vi "SMTP Email Convert Recipients UTF-8.vi"(0 "recipients":string[](array[string]), 1 "error in":errorcluster) -> (2 "convertible recipients":string[](array[string]), 3 "unconvertible recipients":string[](array[string]), 4 "error out":errorcluster)   [LabVIEW 2011, in "NewNI_SMTPEmail.lvlib"]
doc: "Converts array of recipients in system current charset to UTF-8. Returns an error if error passed in, otherwise passes list of convertable and unconvertable recipient entries."
uses:
  NewNI_SMTPEmail.lvlib
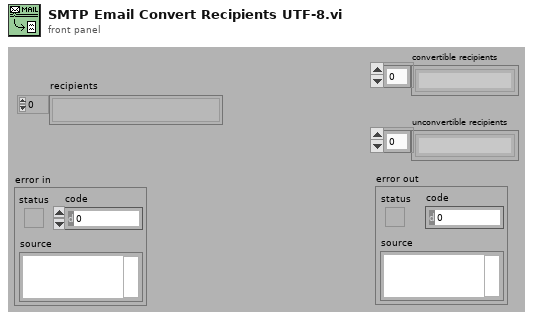
[diagram p1: front panel]
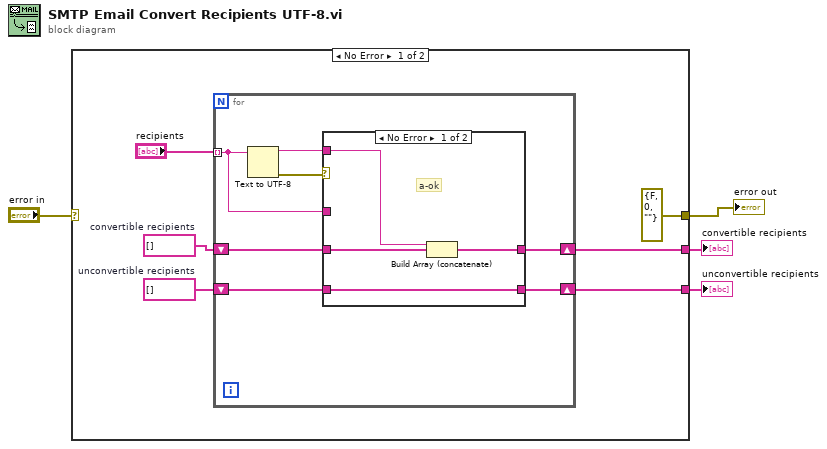
[diagram p0: block diagram]
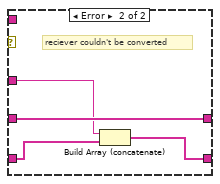
[diagram p2: hidden frame]
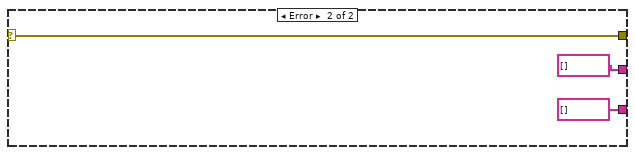
[diagram p3: hidden frame]
diagram:
  n1 = case shown="No Error" "error in" {
    selector: "error in" -> [_ w28]
    tunnel: [errorcluster {"status"=FALSE, "code"=0, "source"=""} ("error IO") w28] -> w3
    tunnel: [w7 string[] [] ("unconvertible recipients")] -> w2
    tunnel: [w6 string[] [] ("convertible recipients")] -> w1
    frame No Error {
      w8 = string[] []  # unconvertible recipients
      w9 = string[] []  # convertible recipients
      n2 = for {
        tunnel: "recipients" -> [w11] mode=indexing
        shift-right: [w14] -> w6
        shift-left: w9 -> [w15]
        shift-right: [w12] -> w7
        shift-left: w8 -> [w13]
        n3 = Text to UTF-8(11:w11) -> (0:w17:errorcluster, 3:w16:string)  [unwired: 1 out]
        n4 = case shown="No Error" w17 {
          tunnel: w16 -> [w21 _]
          tunnel: w15 -> [w20 w25]
          tunnel: [w19 w25] -> w14
          tunnel: w13 -> [w18 w23]
          tunnel: [w18 w22] -> w12
          tunnel: w11 -> [_ w24]
          frame No Error {
            # "a-ok"
            n5 = Build Array (concatenate)(w21, w20) -> (w19:string[])
          }
          frame Error {
            # "reciever couldn't be converted"
            n6 = Build Array (concatenate)(w24, w23) -> (w22:string[])
          }
        }
      }
    }
    frame Error {
    }
  }
  "error out" <- w3
  "unconvertible recipients" <- w2
  "convertible recipients" <- w1
